vi "Write DAQmx Configuration.vi"(8 "error in (no error)":errorcluster, 10 "Configuration":T1 {"input configuration" items=["Default"=-1, "RSE"=10083, "NRSE"=10078, "Differential"=10106, "Pseudodifferential"=12529]; "Rate" format="%#_6pHz"; "Post-trigger duration" format="%#_6ps"; "Pre-trigger duration" format="%#_6ps"; "Range" format="%#_6pV"}, 11 "DAQmx Recorder in":refnum<class "DAQmx Recorder.lvclass">) -> (0 "error out":errorcluster, 3 "DAQmx Recorder out":refnum<class "DAQmx Recorder.lvclass">)   [LabVIEW 2015]
uses:
  DAQmx Recorder.lvclass
  NHMFL_Core/Libraries/NI-DAQ/DAQmx Digitizer/DAQmx Digitizer Configuration.ctl
  Measure_core/Measure Object/Measure Object.lvclass/Measure Object.ctl
  Measure_core/Measure Object/Write Configuration.vi
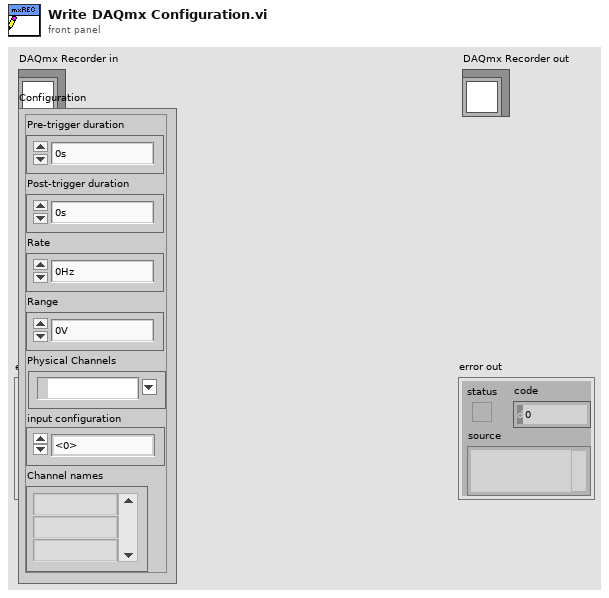
[diagram p1: front panel]
types:
  T1 = typedef "DAQmx Digitizer Configuration.ctl" = cluster{"Pre-trigger duration":dbl, "Post-trigger duration":dbl, "Rate":dbl, "Range":dbl, "Physical Channels":tag, "input configuration":i32, "Channel names":string[]}
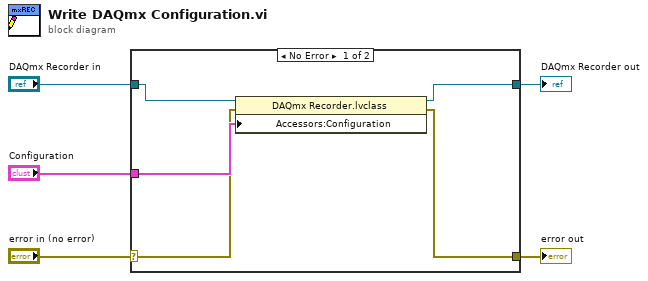
[diagram p0: block diagram]
diagram:
  n1 = case shown="No Error" "error in (no error)" {
    selector: "error in (no error)" -> [w7 w11]
    tunnel: [w6 w11] -> w4
    tunnel: [w8 w12] -> w2
    tunnel: "DAQmx Recorder in" -> [w9 w12]
    tunnel: "Configuration" -> [w10 _]
    frame No Error {
      n2 = property class="DAQmx Recorder.lvclass"(reference=w9, error in=w7, "Accessors:Configuration"=w10) -> (reference out=w8:refnum<class "DAQmx Recorder.lvclass">, error out=w6:errorcluster)
    }
    frame Error {
    }
  }
  "error out" <- w4
  "DAQmx Recorder out" <- w2
